vi "HXG2_Air Flow Calc_REV2.vi"(0 "1\" Nozzle":bool, 1 "0.75\" Nozzle":bool, 2 "2.5inWC Sensor?":bool, 5 "1.25\" Nozzle":bool, 7 "1.5\" Nozzle":bool, 9 "AFM In Temp":dbl, 11 "error in (no error)":errorcluster, 12 "AFM In Hum":dbl, 13 "Nozzle DP":dbl, 14 "Barometric":dbl) -> (4 "CFM Nozzles":dbl, 6 "MinACFM":dbl, 8 "MaxACFM":dbl, 15 "error out":errorcluster)   [LabVIEW 2010]
doc: "This VI will calculate volumetric flow and provide the max and min flows that can be achieved with a particular nozzle combination."
panel:
  out "output variable":i16
  out "Rho per ASHRAE":dbl
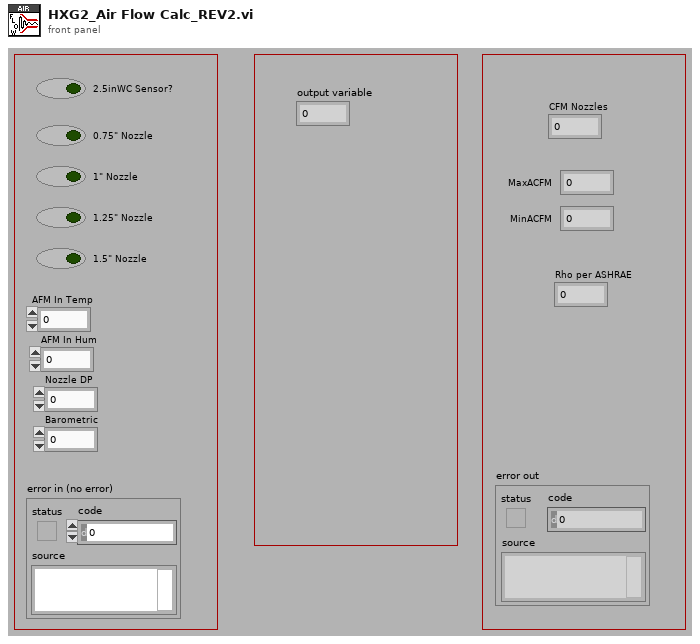
[diagram p1: front panel]
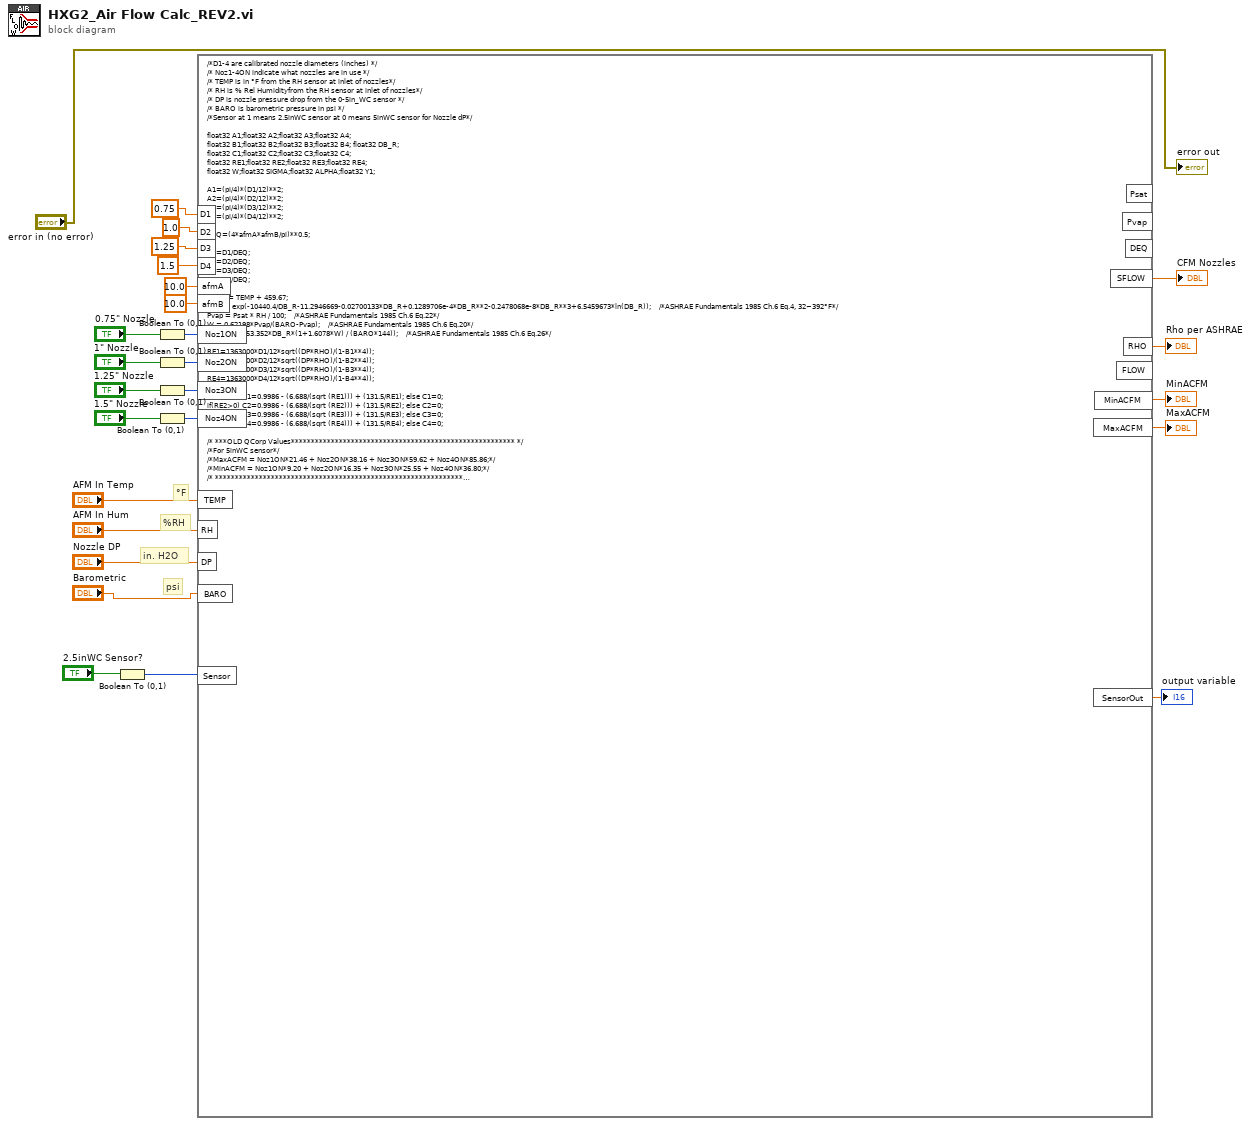
[diagram p0: block diagram]
diagram:
  # "in. H2O"
  # "%RH"
  # "°F"
  # "psi"
  n1 = Boolean To (0,1)(Boolean="2.5inWC Sensor?") -> (0, 1=w3:i16)
  n2 = Boolean To (0,1)(Boolean="0.75\" Nozzle") -> (0, 1=w19:i16)
  n3 = Boolean To (0,1)(Boolean="1\" Nozzle") -> (0, 1=w21:i16)
  n4 = Boolean To (0,1)(Boolean="1.25\" Nozzle") -> (0, 1=w22:i16)
  n5 = Boolean To (0,1)(Boolean="1.5\" Nozzle") -> (0, 1=w20:i16)
  n6 = formula code="/*D1-4 are calibrated nozzle diameters (inches) */\n/* Noz1-4ON indicate what nozzles are in use */\n/* TEMP is in °F from the RH sensor at inlet of nozzles*/\n/* RH is % Rel Humidityfrom the RH sensor at inlet of nozzles*/\n/* DP is nozzle pressure drop from the 0-5in_WC sensor */\n/* BARO is barometric pressure in psi */ \n/*Sensor at 1 means 2.5inWC sensor at 0 means 5inWC sensor for Nozzle dP*/\n\nfloat32 A1;float32 A2;float32 A3;float32 A4;\nfloat32 B1;float32 B2;float32 B3;float32 B4; float32 DB_R;\nfloat32 C1;float32 C2;float32 C3;float32 C4;\nfloat32 RE1;float32 RE2;float32 RE3;float32 RE4;\nfloat32 W;float32 SIGMA;float32 ALPHA;float32 Y1; \n\nA1=(pi/4)*(D1/12)**2;\nA2=(pi/4)*(D2/12)**2;\nA3=(pi/4)*(D3/12)**2;\nA4=(pi/4)*(D4/12)**2;\n\nDEQ=(4*afmA*afmB/pi)**0.5;\n\nB1=D1/DEQ;\nB2=D2/DEQ;\nB3=D3/DEQ;\nB4=D4/DEQ;\n\nDB_R = TEMP + 459.67;\nPsat = exp(-10440.4/DB_R-11.2946669-0.02700133*DB_R+0.1289706e-4*DB_R**2-0.2478068e-8*DB_R**3+6.5459673*ln(DB_R));    /*ASHRAE Fundamentals 1985 Ch.6 Eq.4, 32~392°F*/\nPvap = Psat * RH / 100;    /*ASHRAE Fundamentals 1985 Ch.6 Eq.22*/\nW = 0.62198*Pvap/(BARO-Pvap);    /*ASHRAE Fundamentals 1985 Ch.6 Eq.20*/\nRHO = 1 / (53.352*DB_R*(1+1.6078*W) / (BARO*144));    /*ASHRAE Fundamentals 1985 Ch.6 Eq.26*/\n\nRE1=1363000*D1/12*sqrt((DP*RHO)/(1-B1**4));\nRE2=1363000*D2/12*sqrt((DP*RHO)/(1-B2**4));\nRE3=1363000*D3/12*sqrt((DP*RHO)/(1-B3**4));\nRE4=1363000*D4/12*sqrt((DP*RHO)/(1-B4**4));\n\nif(RE1>0) C1=0.9986 - (6.688/(sqrt (RE1))) + (131.5/RE1); else C1=0;\nif(RE2>0) C2=0.9986 - (6.688/(sqrt (RE2))) + (131.5/RE2); else C2=0;\nif(RE3>0) C3=0.9986 - (6.688/(sqrt (RE3))) + (131.5/RE3); else C3=0;\nif(RE4>0) C4=0.9986 - (6.688/(sqrt (RE4))) + (131.5/RE4); else C4=0;\n\n/* ***OLD QCorp Values******************************************************** */\n/*For 5inWC sensor*/\n/*MaxACFM = Noz1ON*21.46 + Noz2ON*38.16 + Noz3ON*59.62 + Noz4ON*85.86;*/\n/*MinACFM = Noz1ON*9.20 + Noz2ON*16.35 + Noz3ON*25.55 + Noz4ON*36.80;*/\n/* **************************************************************************** */\nSensorOut = Sensor;\n/*For 2.5inWC sensor*/\n/*Max and Min flow calculated from 2.45 and 0.35inWC limit pressures*/\n\nif(Sensor==1) {\nMaxACFM = Noz1ON*18.5 + Noz2ON*33 + Noz3ON*51.7 + Noz4ON*74.7;\nMinACFM = Noz1ON*6.9 + Noz2ON*12.3 + Noz3ON*19.3 + Noz4ON*27.9;\n}\n/*For 5inWC sensor*/\nelse {\nMaxACFM = Noz1ON*25.11 + Noz2ON*44.8 + Noz3ON*70.17 + Noz4ON*101.24;\nMinACFM = Noz1ON*11.8 + Noz2ON*21.0 + Noz3ON*32.9 + Noz4ON*47.5;\n}\n\n/* **************************************************************************** */\n\nSIGMA = Noz1ON*C1*A1 + Noz2ON*C2*A2 + Noz3ON*C3*A3 + Noz4ON*C4*A4;\nALPHA = (BARO-DP*.036)/BARO;\nY1 = 1-(0.548+.71*B4**4)*(1-ALPHA);\nif (DP>0) FLOW = 1096*Y1*((DP/RHO)**.5)*SIGMA; else FLOW=0;\nSFLOW = FLOW*(RHO/0.075);"("D2"=1.0 ("input variable"), "D4"=1.5 ("input variable"), "D1"=0.75 ("input variable"), "D3"=1.25 ("input variable"), "DP"="Nozzle DP", "BARO"="Barometric", "TEMP"="AFM In Temp", "RH"="AFM In Hum", "afmA"=10.0 ("input variable"), "afmB"=10.0 ("input variable"), "Noz1ON"=w19, "Noz2ON"=w21, "Noz3ON"=w22, "Noz4ON"=w20, "Sensor"=w3) -> ("SFLOW"=→"CFM Nozzles":dbl, "RHO"=→"Rho per ASHRAE":dbl, "MaxACFM"=→"MaxACFM":dbl, "MinACFM"=→"MinACFM":dbl, "SensorOut"=→"output variable":dbl)  [unwired: 4 out]
  "error out" <- "error in (no error)"
